vi "HMF2500 Set Ext Reference.vi"(8 "error in (no error)":errorcluster, 10 "Uset Ext Ref Clock (False)":bool, 11 "VISA in":refnum<visa-resource-name>) -> (0 "error out":errorcluster, 3 "VISA out":refnum<visa-resource-name>)   [LabVIEW 2020, in "AWG.lvlib"]
doc: "Enable/disable external reference clock 10MHz."
uses:
  AWG.lvlib
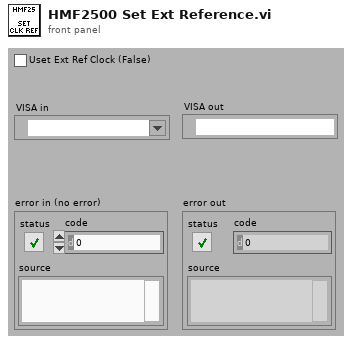
[diagram p1: front panel]
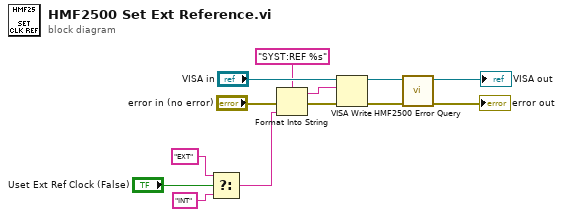
[diagram p0: block diagram]
diagram:
  n1 = Select(t="EXT", s="Uset Ext Ref Clock (False)", f="INT") -> (s? t:f=w6:string)
  n2 = Format Into String(format string="SYST:REF %s", error in="error in (no error)", w6) -> (resulting string=w11:string, error out=w12:errorcluster)  [unwired: 1 in]
  n3 = VISA Write(VISA resource name="VISA in", write buffer=w11, error in (no error)=w12) -> (VISA resource name out=w3:refnum<visa-resource-name>, error out=w4:errorcluster)  [unwired: 1 out]
  n4 = call "HMF2500 Error Query.vi"("error in (no error)"=w4, "VISA resource name"=w3) -> ("error out"=→"error out":errorcluster, "VISA resource name out"=→"VISA out":refnum<visa-resource-name>)  [unwired: 6 in, 2 out]
